vi "initialize runtime lines.vi"(0 "Shared Memory runtime in":refnum<class "Shared Memory runtime.lvclass">, 5 "shared memory name":string, 7 "Lines":T5[](array[typedef]), 9 "data allocations in":T1, 11 "error in (no error)":errorcluster, 12 "channel classification":T4) -> (4 "Shared Memory runtime out":refnum<class "Shared Memory runtime.lvclass">, 15 "error out":errorcluster)   [LabVIEW 2014, in "Shared Memory runtime.lvclass"]
uses:
  Shared Memory runtime.lvclass
  configuration/Line.ctl
  <vilib>/NI/Tag Bus Module Framework/channel/TBM channel.lvclass
  <vilib>/NI/Tag Bus Module Framework/channel/channel classification.ctl
  <vilib>/NI/Tag Bus Module Framework/channel/data tables.ctl
  <vilib>/NI/Tag Bus/dictionary/data dictionary.lvclass
  <vilib>/NI/Tag Bus/dictionary table pair.ctl
  <vilib>/NI/Tag Bus/table/data table.ctl
  <vilib>/NI/Tag Bus/tag/tag descriptor.lvclass/tag descriptor.ctl
  Shared Memory runtime.lvclass/Shared Memory runtime.ctl
  <vilib>/NI/Tag Bus/tag/read tag name.vi
  <vilib>/NI/Tag Bus/dictionary/locate tag.vi
  <vilib>/NI/Tag Bus/tag/tag descriptor.lvclass
  configuration/Shared Memory configuration.lvclass
  <vilib>/NI/Tag Bus/table/data table.lvlib
  <vilib>/NI/Tag Bus/tag bus.lvlib
types:
  T1 = typedef "TBM channel.lvclass/data tables.ctl" = cluster{"input data":T2, "processing parameter":T2, "processing result":T2, "output data":T2}
  T2 = typedef "tag bus.lvlib/dictionary table pair.ctl" = cluster{"data dictionary":refnum<class "data dictionary.lvclass">, "data table":T3}
  T3 = typedef "tag bus.lvlib/data table.lvlib/data table.ctl" = cluster{"Double":dbl[], "Single":sgl[], "I64":i64[], "I32":i32[], "I16":i16[], "I8":i8[], "U64":u64[], "U32":u32[], "U16":u16[], "U8":u8[], "Boolean":bool[], "String":string[], "Array of Double":cluster{"DBL Array":dbl[]}[], "Array of Single":cluster{"SGL Array":sgl[]}[], "Array of I64":cluster{"I64 Array":i64[]}[], "Array of I32":cluster{"I32 Array":i32[]}[], "Array of I16":cluster{"I16 Array":i16[]}[], "Array of I8":cluster{"I8 Array":i8[]}[], "Array of U64":cluster{"U64 Array":u64[]}[], "Array of U32":cluster{"U32 Array":u32[]}[], "Array of U16":cluster{"U16 Array":u16[]}[], "Array of U8":cluster{"U8 Array":u8[]}[], "Array of Boolean":cluster{"Boolean Array":bool[]}[], "Array of String":cluster{"String Array":string[]}[]}
  T4 = typedef "TBM channel.lvclass/channel classification.ctl" = enum16{"input data", "output data", "processing parameter", "processing result"}
  T5 = typedef "Shared Memory configuration.lvclass/Line.ctl" = cluster{"channel":refnum<class "TBM channel.lvclass">}
  T6 = typedef "tag bus.lvlib/tag descriptor.lvclass/Data Type.ctl" = enum16{"Double", "Single", "I64", "I32", "I16", "I8", "U64", "U32", "U16", "U8", "Boolean", "String", "Array of Double", "Array of Single", "Array of I64", "Array of I32", "Array of I16", "Array of I8", "Array of U64", "Array of U32", "Array of U16", "Array of U8", "Array of Boolean", "Array of String"}
  T7 = typedef "Shared Memory runtime.lvclass/channel runtime.ctl" = cluster{"channel classification":T4, "data type":T6, "pointer to shared memory":u64, "number of elements":u64, "data dictionary index":cluster{i32[]}, "shared memory":T8, "first tag index":i32, "sequential tags?":bool}
  T8 = typedef "Linux RT IPC.lvlib/Shared Memory.lvlib/reference.ctl" = refnum<data-value>
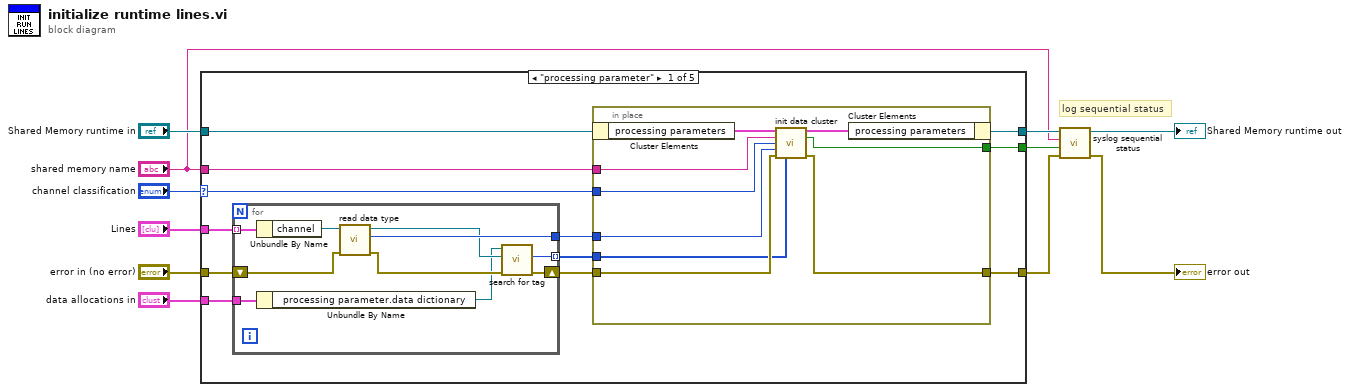
[diagram p0: block diagram]
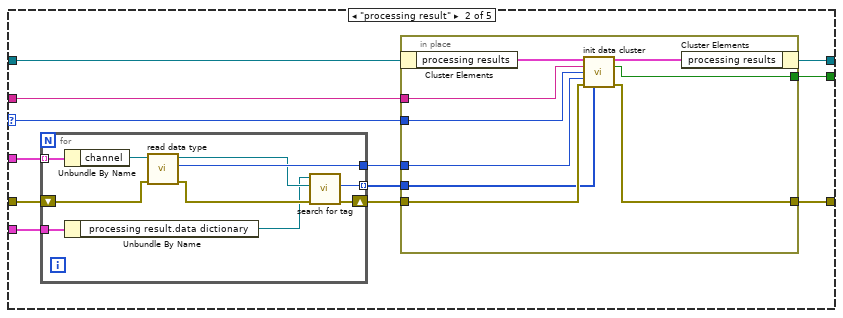
[diagram p2: hidden frame]
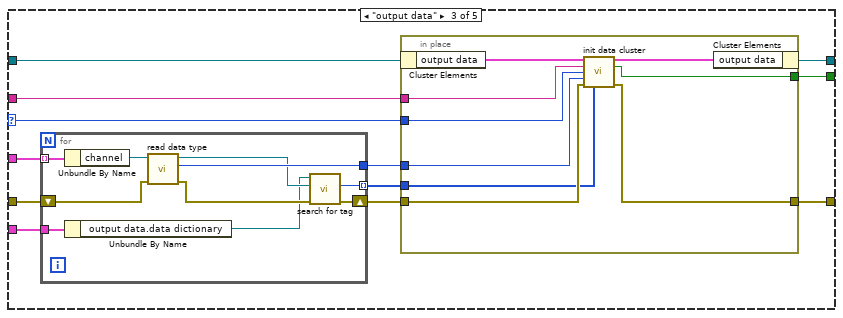
[diagram p3: hidden frame]
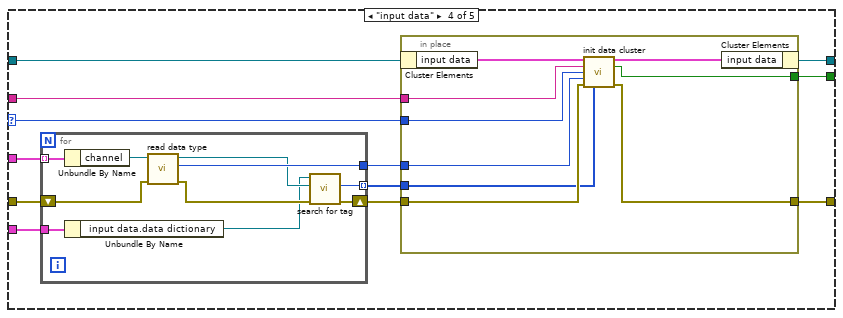
[diagram p4: hidden frame]
diagram:
  # "log sequential status"
  n1 = case shown="\"processing parameter\"" "channel classification" {
    selector: "channel classification" -> [w20 w51 w82 w113 _]
    tunnel: "data allocations in" -> [w23 w54 w85 w116 _]
    tunnel: "error in (no error)" -> [w15 w46 w77 w108 w136]
    tunnel: "Shared Memory runtime in" -> [w22 w53 w84 w115 w137]
    tunnel: [w21 w52 w83 w114 w137] -> w6
    tunnel: "shared memory name" -> [w16 w47 w78 w109 _]
    tunnel: [w17 w48 w79 w110 w136] -> w4
    tunnel: "Lines" -> [w13 w44 w75 w106 _]
    tunnel: [w12 w43 w74 w105 _] -> w1
    frame "processing parameter" {
      n2 = for {
        tunnel: w23 -> [w25]
        tunnel: [w33] -> w19 mode=indexing
        tunnel: [w31] -> w14
        shift-right: [w28] -> w18
        shift-left: w15 -> [w32]
        tunnel: w13 -> [w27] mode=indexing
        n3 = Unbundle By Name(w27) -> ("channel"=w26:refnum<class "TBM channel.lvclass">)
        n4 = Unbundle By Name(w25) -> ("processing parameter.data dictionary"=w24:refnum<class "data dictionary.lvclass">)
        n5 = call <vilib>:"read data type.vi"("error in"=w32, "system tag in"=w26) -> ("error out"=w29:errorcluster, "data type"=w31:T6, "system tag out"=w30:refnum<class "TBM channel.lvclass">)  [unwired: 7 in]
        n6 = call <vilib>:"search for tag.vi"("error in"=w29, "system tag"=w30, "data dictionary in"=w24) -> ("error out"=w28:errorcluster, "index"=w33:i32)  [unwired: 6 in, 1 out]
      }
      n7 = in-place {
        in-place-border: w19 -> [w35]
        in-place-border: w14 -> [w37]
        in-place-border: w16 -> [w39]
        in-place-border: w20 -> [w38]
        in-place-border: w18 -> [w36]
        in-place-border: [w40] -> w17
        in-place-border: [w34] -> w12
        n8 = in-place-cluster #1(w22) -> ("processing parameters"=w42:T7[])
        n9 = call "init data cluster.vi"("data clusters in"=w42, "shared memory name"=w39, "channel classification"=w38, "data type"=w37, "error in"=w36, "index"=w35) -> ("data clusters out"=w41:T7[], "sequential tags?"=w34:bool, "error out"=w40:errorcluster)  [unwired: 7 in]
        n10 = in-place-cluster #1("processing parameters"=w41) -> (w21:refnum<class "Shared Memory runtime.lvclass">)
      }
    }
    frame "processing result" {
      n11 = for {
        tunnel: w54 -> [w56]
        tunnel: [w64] -> w50 mode=indexing
        tunnel: [w62] -> w45
        shift-right: [w59] -> w49
        shift-left: w46 -> [w63]
        tunnel: w44 -> [w58] mode=indexing
        n12 = Unbundle By Name(w58) -> ("channel"=w57:refnum<class "TBM channel.lvclass">)
        n13 = Unbundle By Name(w56) -> ("processing result.data dictionary"=w55:refnum<class "data dictionary.lvclass">)
        n14 = call <vilib>:"read data type.vi"("error in"=w63, "system tag in"=w57) -> ("error out"=w60:errorcluster, "data type"=w62:T6, "system tag out"=w61:refnum<class "TBM channel.lvclass">)  [unwired: 7 in]
        n15 = call <vilib>:"search for tag.vi"("error in"=w60, "system tag"=w61, "data dictionary in"=w55) -> ("error out"=w59:errorcluster, "index"=w64:i32)  [unwired: 6 in, 1 out]
      }
      n16 = in-place {
        in-place-border: w50 -> [w66]
        in-place-border: w45 -> [w68]
        in-place-border: w47 -> [w70]
        in-place-border: w51 -> [w69]
        in-place-border: w49 -> [w67]
        in-place-border: [w71] -> w48
        in-place-border: [w65] -> w43
        n17 = in-place-cluster #2(w53) -> ("processing results"=w73:T7[])
        n18 = call "init data cluster.vi"("data clusters in"=w73, "shared memory name"=w70, "channel classification"=w69, "data type"=w68, "error in"=w67, "index"=w66) -> ("data clusters out"=w72:T7[], "sequential tags?"=w65:bool, "error out"=w71:errorcluster)  [unwired: 7 in]
        n19 = in-place-cluster #2("processing results"=w72) -> (w52:refnum<class "Shared Memory runtime.lvclass">)
      }
    }
    frame "output data" {
      n20 = for {
        tunnel: w85 -> [w87]
        tunnel: [w95] -> w81 mode=indexing
        tunnel: [w93] -> w76
        shift-right: [w90] -> w80
        shift-left: w77 -> [w94]
        tunnel: w75 -> [w89] mode=indexing
        n21 = Unbundle By Name(w89) -> ("channel"=w88:refnum<class "TBM channel.lvclass">)
        n22 = Unbundle By Name(w87) -> ("output data.data dictionary"=w86:refnum<class "data dictionary.lvclass">)
        n23 = call <vilib>:"read data type.vi"("error in"=w94, "system tag in"=w88) -> ("error out"=w91:errorcluster, "data type"=w93:T6, "system tag out"=w92:refnum<class "TBM channel.lvclass">)  [unwired: 7 in]
        n24 = call <vilib>:"search for tag.vi"("error in"=w91, "system tag"=w92, "data dictionary in"=w86) -> ("error out"=w90:errorcluster, "index"=w95:i32)  [unwired: 6 in, 1 out]
      }
      n25 = in-place {
        in-place-border: w81 -> [w97]
        in-place-border: w76 -> [w99]
        in-place-border: w78 -> [w101]
        in-place-border: w82 -> [w100]
        in-place-border: w80 -> [w98]
        in-place-border: [w102] -> w79
        in-place-border: [w96] -> w74
        n26 = in-place-cluster #3(w84) -> ("output data"=w104:T7[])
        n27 = call "init data cluster.vi"("data clusters in"=w104, "shared memory name"=w101, "channel classification"=w100, "data type"=w99, "error in"=w98, "index"=w97) -> ("data clusters out"=w103:T7[], "sequential tags?"=w96:bool, "error out"=w102:errorcluster)  [unwired: 7 in]
        n28 = in-place-cluster #3("output data"=w103) -> (w83:refnum<class "Shared Memory runtime.lvclass">)
      }
    }
    frame "input data" {
      n29 = for {
        tunnel: w116 -> [w118]
        tunnel: [w126] -> w112 mode=indexing
        tunnel: [w124] -> w107
        shift-right: [w121] -> w111
        shift-left: w108 -> [w125]
        tunnel: w106 -> [w120] mode=indexing
        n30 = Unbundle By Name(w120) -> ("channel"=w119:refnum<class "TBM channel.lvclass">)
        n31 = Unbundle By Name(w118) -> ("input data.data dictionary"=w117:refnum<class "data dictionary.lvclass">)
        n32 = call <vilib>:"read data type.vi"("error in"=w125, "system tag in"=w119) -> ("error out"=w122:errorcluster, "data type"=w124:T6, "system tag out"=w123:refnum<class "TBM channel.lvclass">)  [unwired: 7 in]
        n33 = call <vilib>:"search for tag.vi"("error in"=w122, "system tag"=w123, "data dictionary in"=w117) -> ("error out"=w121:errorcluster, "index"=w126:i32)  [unwired: 6 in, 1 out]
      }
      n34 = in-place {
        in-place-border: w112 -> [w128]
        in-place-border: w107 -> [w130]
        in-place-border: w109 -> [w132]
        in-place-border: w113 -> [w131]
        in-place-border: w111 -> [w129]
        in-place-border: [w133] -> w110
        in-place-border: [w127] -> w105
        n35 = in-place-cluster #4(w115) -> ("input data"=w135:T7[])
        n36 = call "init data cluster.vi"("data clusters in"=w135, "shared memory name"=w132, "channel classification"=w131, "data type"=w130, "error in"=w129, "index"=w128) -> ("data clusters out"=w134:T7[], "sequential tags?"=w127:bool, "error out"=w133:errorcluster)  [unwired: 7 in]
        n37 = in-place-cluster #4("input data"=w134) -> (w114:refnum<class "Shared Memory runtime.lvclass">)
      }
    }
    frame Default {
    }
  }
  n38 = call "syslog sequential status.vi"("error in (no error)"=w4, "sequential tags?"=w1, "shared memory name"="shared memory name", "shared memory runtime in"=w6) -> ("error out"=→"error out":errorcluster, "shared memory runtime out"=→"Shared Memory runtime out":refnum<class "Shared Memory runtime.lvclass">)  [unwired: 6 in]
